vi "Write Value.vi"(8 "error in (no error)":errorcluster, 10 "value":variant, 11 "NT Base in":refnum<class "NT Base.lvclass">) -> (0 "error out":errorcluster, 3 "NT Base out":refnum<class "NT Base.lvclass">)   [LabVIEW 2020, in "PV Access.lvlib" / "PV Data.lvlib" / "NT Base.lvclass"]
uses:
  NT Base.lvclass
  NT Base.lvclass/NT Base.ctl
  <vilib>/ErrorRing/Error Ring.xnode
  PV Data.lvlib
  <vilib>/Utility/error.llb/Error Cluster From Error Code.vi
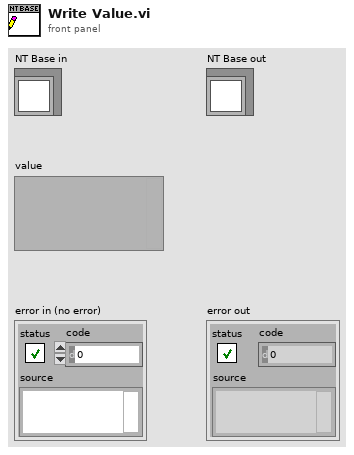
[diagram p1: front panel]
types:
  T1 = typedef "PV Access.lvlib/PV Data.lvlib/Type Code.ctl" = enum8{"Null", "Bool", "BoolA", "Int8", "Int8A", "Int16", "Int16A", "Int32", "Int32A", "Int64", "Int64A", "UInt8", "UInt8A", "UInt16", "UInt16A", "UInt32", "UInt32A", "UInt64", "UInt64A", "Float32", "Float32A", "Float64", "Float64A", "String", "StringA", "Struct", "StructA", "Union", "UnionA", "Any", "AnyA"}
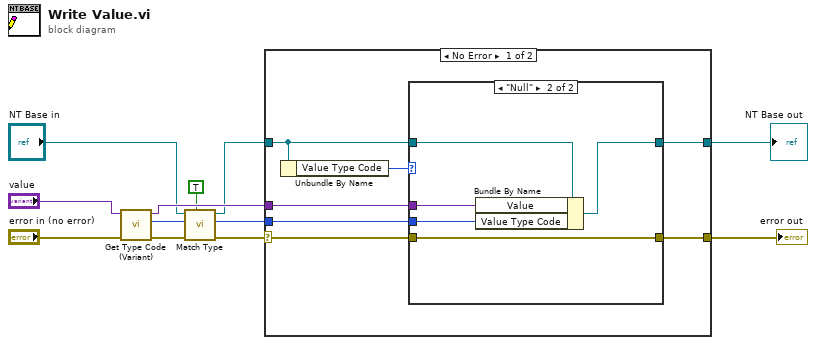
[diagram p0: block diagram]
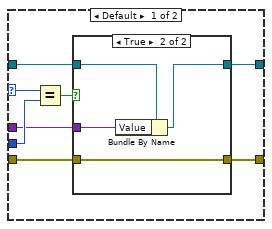
[diagram p2: hidden frame]
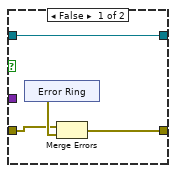
[diagram p3: hidden frame]
diagram:
  n1 = call "Get Type Code (Variant).vi"("error in (no error)"="error in (no error)", "value"="value") -> ("error out"=w5:errorcluster, "type code"=w7:T1, "value dup"=w8:variant)  [unwired: 5 in]
  n2 = call-dynamic "Match Type.vi"("raise for mismatch?"=TRUE, "error in (no error)"=w5, "type code"=w7, "NT Base in"="NT Base in") -> ("error out"=w4:errorcluster, "type code out"=w6:T1, "NT Base out"=w2:refnum<class "NT Base.lvclass">)  [unwired: 4 in, 1 out]
  n3 = case shown="No Error" w4 {
    selector: w4 -> [w15 w46]
    tunnel: [w19 w46] -> w11
    tunnel: [w18 w45] -> w10
    tunnel: w8 -> [w17 _]
    tunnel: w6 -> [w16 _]
    tunnel: w2 -> [w14 w45]
    frame No Error {
      n4 = Unbundle By Name(w14) -> ("Value Type Code"=w13:T1)
      n5 = case shown="\"Null\"" w13 {
        selector: w13 -> [w27 _]
        tunnel: w16 -> [w26 w41]
        tunnel: w15 -> [w25 w44]
        tunnel: w17 -> [w20 w40]
        tunnel: [w24 w44] -> w19
        tunnel: w14 -> [w22 w43]
        tunnel: [w21 w42] -> w18
        frame Default {
          n6 = Equal?(x=w27, y=w26) -> (x = y?=w23:bool)
          n7 = case shown="True" w23 {
            tunnel: w25 -> [w30 w39]
            tunnel: [w29 w39] -> w24
            tunnel: w22 -> [w28 w38]
            tunnel: [w28 w37] -> w21
            tunnel: w20 -> [_ w36]
            frame False {
              n8 = xnode "Error Ring"() -> ("error out"=w31:errorcluster)
              n9 = Merge Errors(w30, w31) -> (w29:errorcluster)
            }
            frame True {
              n10 = Bundle By Name(cluster=w38, "Value"=w36) -> (w37:refnum<class "NT Base.lvclass">)
            }
          }
        }
        frame "Null" {
          n11 = Bundle By Name(cluster=w43, "Value"=w40, "Value Type Code"=w41) -> (w42:refnum<class "NT Base.lvclass">)
        }
      }
    }
    frame Error {
    }
  }
  "error out" <- w11
  "NT Base out" <- w10
